vi "DAQ-ClearDevice.vi"(0 "DAQ Device IN":T1) -> ()   [LabVIEW 2010]
uses:
  <vilib>/Utility/error.llb/DialogType.ctl
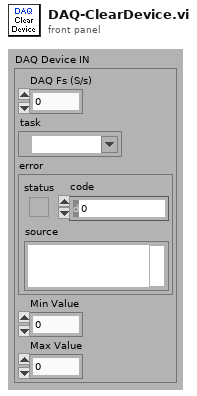
[diagram p1: front panel]
types:
  T1 = cluster{"DAQ Fs (S/s)":dbl, "task":refnum<k21>, "error":errorcluster, "Min Value":dbl, "Max Value":dbl}
  T2 = typedef "DialogType.ctl" = u16
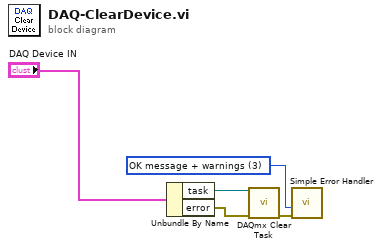
[diagram p0: block diagram]
diagram:
  w2 = T2 3 items=["no dialog", "OK message", "continue or stop message", "OK message + warnings", "continue/stop + warnings"] ("type of dialog (OK msg:1)")
  n1 = Unbundle By Name("DAQ Device IN") -> ("task"=w4:refnum<k21>, "error"=w5:errorcluster)
  n2 = call <vilib>:"DAQmx Clear Task.vi"("task in"=w4, "error in"=w5) -> ("error out"=w1:errorcluster)  [unwired: 13 in]
  n3 = call <vilib>:"Simple Error Handler.vi"("type of dialog (OK msg:1)"=w2, "error in (no error)"=w1) -> ()  [unwired: 3 in, 5 out]
